vi "快速逼近索引法.vi"(8 "数值":dbl format="%#_13g", 11 "数组":dbl[](array[numeric])) -> (2 "最近索引":i32)   [LabVIEW 2017]
doc: "功能：获取“数值”在非空“顺序数组”中最近的索引。\n如果数组为空，返回索引 -1。"
panel:
  out "s? t:f":enum16{"顺序", "逆序"}(ring)
  # "功能：获取“数值”在非空“顺序数组”中最近的索引"
  # "注：数组不可为空，否则死循环！！"
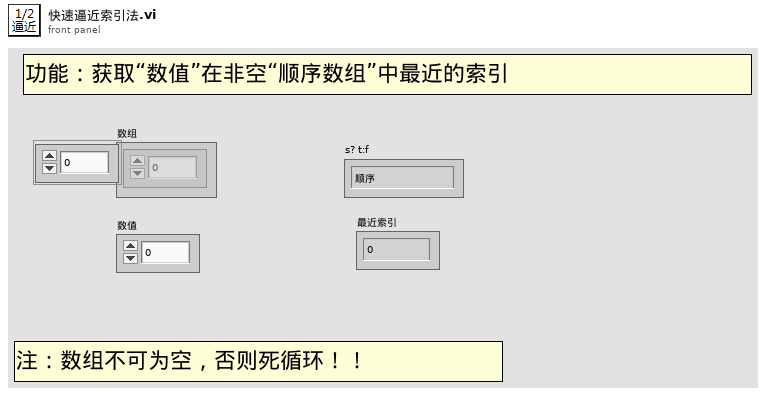
[diagram p1: front panel]
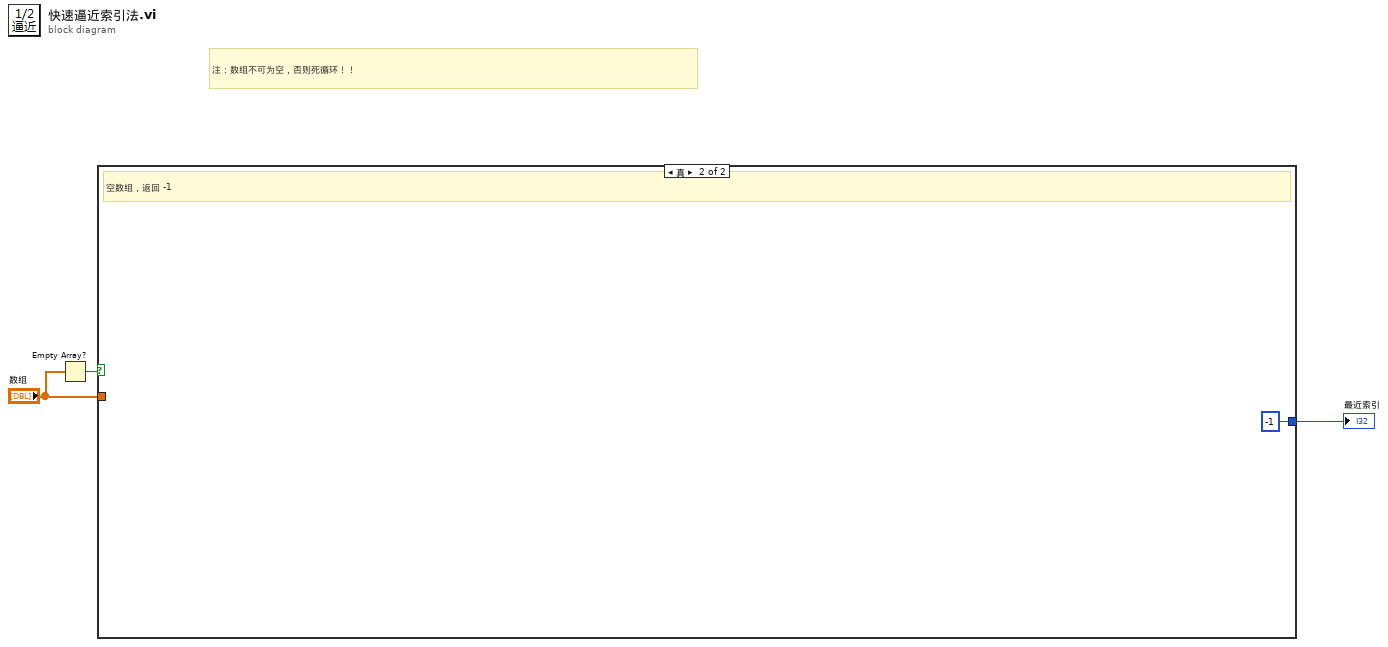
[diagram p0: block diagram]
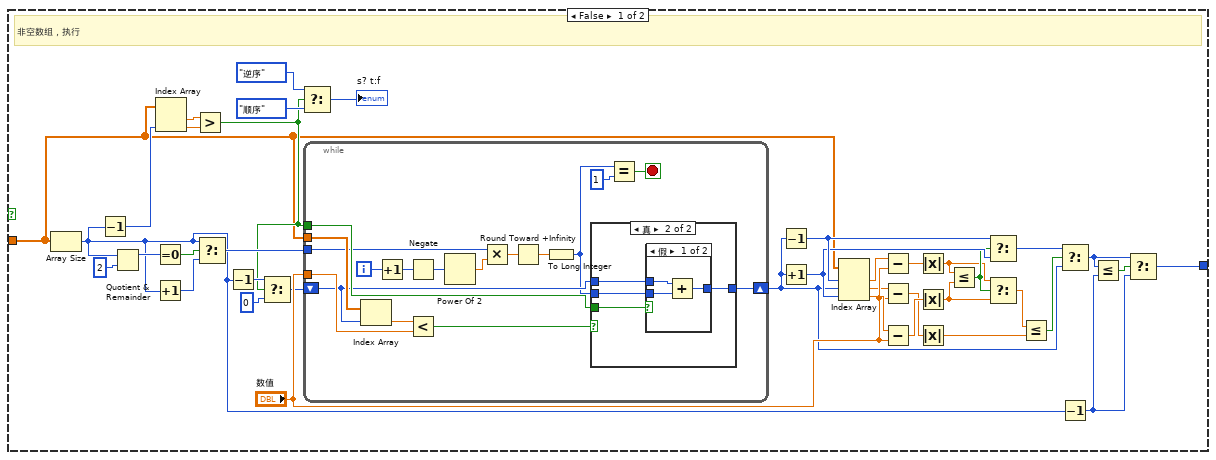
[diagram p2: hidden frame]
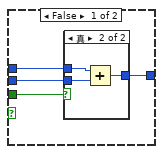
[diagram p3: hidden frame]
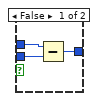
[diagram p4: hidden frame]
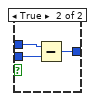
[diagram p5: hidden frame]
diagram:
  # "注：数组不可为空，否则死循环！！"
  n1 = Empty Array?(array="数组") -> (empty?=w1:bool)
  n2 = case shown="真" w1 {
    tunnel: [w25 -1 ("索引")] -> w3
    tunnel: "数组" -> [w4 _]
    frame False {
      # "非空数组，执行"
      n3 = Array Size(array=w4) -> (size(s)=w9:i32)
      n4 = Decrement(x=w9) -> (x-1=w41:i32)
      n5 = Quotient & Remainder(x=w9, y=2) -> (x-y*floor(x/y)=w34:i32)  [unwired: 1 out]
      n6 = Equal To 0?(x=w34) -> (x = 0?=w33:bool)
      n7 = Increment(x=w9) -> (x+1=w32:i32)
      n8 = Index Array(array=w4, index #2=w41) -> (element #1=w39:dbl, element #2=w40:dbl)  [unwired: 1 in]
      n9 = Greater?(x=w39, y=w40) -> (0:w6:bool)
      n10 = Select(t=w9, s=w33, f=w32) -> (s? t:f=w31:i32)
      n11 = Decrement(x=w9) -> (x-1=w8:i32)
      n12 = Select(t=w8, s=w6, f=0 ("索引")) -> (s? t:f=w5:i32)
      n13 = Select(t=enum16{"顺序", "逆序"}."逆序", s=w6, f=enum16{"顺序", "逆序"}."顺序") -> (s? t:f=→"s? t:f":enum16{"顺序", "逆序"})
      n14 = while {
        tunnel: w4 -> [w58]
        tunnel: "数值" -> [w56]
        shift-right: [w51] -> w11
        shift-left: w5 -> [w52]
        tunnel: w31 -> [w44]
        tunnel: w6 -> [w55]
        i -> [w47]
        stop <- w48 stop-if-true
        n15 = Index Array(array=w58, index=w52) -> (element=w57:dbl)
        n16 = Increment(x=w47) -> (x+1=w46:i32)
        n17 = Negate(x=w46) -> (-x=w45:i32)
        n18 = Less?(x=w57, y=w56) -> (x < y?=w54:bool)
        n19 = Power Of 2(x=w45) -> (2^x=w43:dbl)
        n20 = Multiply(x=w44, y=w43) -> (x*y=w42:dbl)
        n21 = Round Toward +Infinity(x=w42) -> (ceil(x): smallest int >= x=w53:dbl)
        n22 = To Long Integer(number=w53) -> (32bit integer=w50:i32)
        n23 = case shown="真" w54 {
          tunnel: w55 -> [w62 w72]
          tunnel: w50 -> [w61 w71]
          tunnel: w52 -> [w60 w70]
          tunnel: [w59 w69] -> w51
          frame False {
            n24 = case shown="真" w62 {
              tunnel: w61 -> [w65 w68]
              tunnel: w60 -> [w64 w67]
              tunnel: [w63 w66] -> w59
              frame False {
                n25 = Subtract(x=w64, y=w65) -> (x-y=w63:i32)
              }
              frame True {
                n26 = Add(x=w67, y=w68) -> (x+y=w66:i32)
              }
            }
          }
          frame True {
            n27 = case shown="假" w72 {
              tunnel: w71 -> [w75 w78]
              tunnel: w70 -> [w74 w77]
              tunnel: [w73 w76] -> w69
              frame False {
                n28 = Add(x=w74, y=w75) -> (x+y=w73:i32)
              }
              frame True {
                n29 = Subtract(x=w77, y=w78) -> (x-y=w76:i32)
              }
            }
          }
        }
        n30 = Equal?(x=w50, y=1) -> (x = y?=w48:bool)
      }
      n31 = Decrement(x=w11) -> (x-1=w20:i32)
      n32 = Increment(x=w11) -> (x+1=w19:i32)
      n33 = Index Array(array=w4, index #1=w20, index #2=w11, index #3=w19) -> (element #1=w30:dbl, element #2=w21:dbl, element #3=w24:dbl)
      n34 = Subtract(x=w30, y="数值") -> (x-y=w28:dbl)
      n35 = Subtract(x=w21, y="数值") -> (x-y=w23:dbl)
      n36 = Subtract(x=w24, y="数值") -> (x-y=w29:dbl)
      n37 = Absolute Value(x=w28) -> (abs(x)=w17:dbl)
      n38 = Absolute Value(x=w29) -> (abs(x)=w16:dbl)
      n39 = Absolute Value(x=w23) -> (abs(x)=w14:dbl)
      n40 = Less Or Equal?(x=w17, y=w16) -> (x <= y?=w18:bool)
      n41 = Select(t=w20, s=w18, f=w19) -> (s? t:f=w12:i32)
      n42 = Select(t=w17, s=w18, f=w16) -> (s? t:f=w15:dbl)
      n43 = Less Or Equal?(x=w15, y=w14) -> (x <= y?=w13:bool)
      n44 = Select(t=w12, s=w13, f=w11) -> (s? t:f=w10:i32)
      n45 = Decrement(x=w9) -> (x-1=w26:i32)
      n46 = Less Or Equal?(x=w10, y=w26) -> (x <= y?=w27:bool)
      n47 = Select(t=w10, s=w27, f=w26) -> (s? t:f=w25:i32)
    }
    frame True {
      # "空数组，返回 -1"
    }
  }
  "最近索引" <- w3
